vi "Build SPA query command substring.vi"(1 "Syntax":T1, 2 "Axes to query":string[](array[string]), 3 "Parameter number":i32[](array[numeric]), 6 "Parameter number (hex)":u32[](array[numeric]) format="%.0x", 7 "Parameter no. format \n(Decimal: FALSE)":bool) -> (14 "Command substring":string, 16 "Number of rows":u32)   [LabVIEW 2020]
doc: "This VI builds an SPA? Command substring. Axes and parameters are combined into a substring. Number of rows is size of Axes to query array. Sub-VI for SPA?.vi and SEP?.vi."
uses:
  Communication.llb/Syntax.ctl
panel:
  # "This vi builds a SPA? command substring. Axes and parameters are combined into a substring, depending on \"Parameter\nno. format\"."
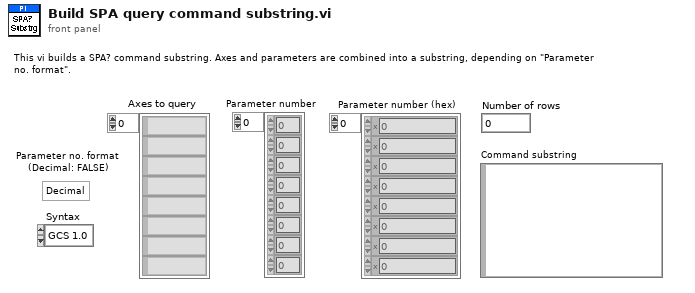
[diagram p1: front panel]
types:
  T1 = typedef "Syntax.ctl" = enum16{"GCS 1.0", "GCS 2.0", "GCS 3.0"}
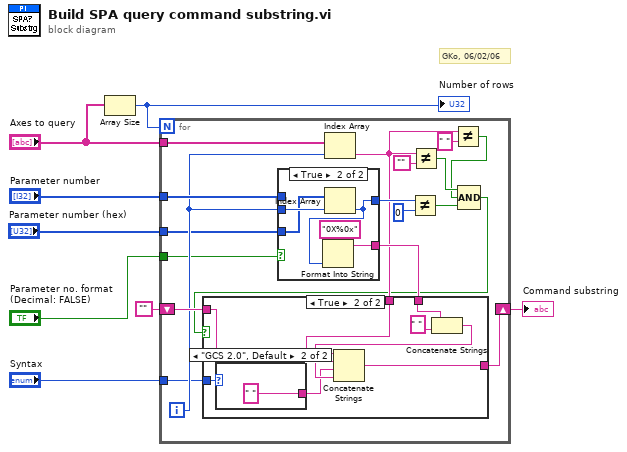
[diagram p0: block diagram]
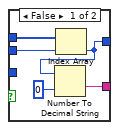
[diagram p2: hidden frame]
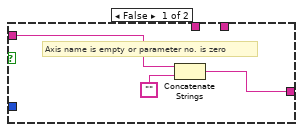
[diagram p3: hidden frame]
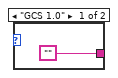
[diagram p4: hidden frame]
diagram:
  # "GKo, 06/02/06"
  n1 = Array Size(array="Axes to query") -> (size(s)=w8:i32)
  "Number of rows" <- w8
  n2 = for {
    N: w8 -> [_]
    shift-right: [w25] -> w6
    shift-left: "" -> [w26]
    tunnel: "Axes to query" -> [w24]
    tunnel: "Parameter number" -> [w23]
    tunnel: "Syntax" -> [w18]
    tunnel: "Parameter no. format \n(Decimal: FALSE)" -> [w10]
    tunnel: "Parameter number (hex)" -> [w9]
    i -> [w22]
    n3 = case shown="True" w10 {
      tunnel: w23 -> [w31 _]
      tunnel: w22 -> [w30 w36]
      tunnel: [w29 w35] -> w21
      tunnel: [w28 w34] -> w19
      tunnel: w9 -> [_ w33]
      frame False {
        n4 = Index Array(array=w31, index=w30) -> (element=w29:i32)
        n5 = Number To Decimal String(number=w29, width (-)=i16 0) -> (decimal integer string=w28:string)
      }
      frame True {
        n6 = Index Array(array=w33, index=w36) -> (element=w35:u32)
        n7 = Format Into String(format string="0X%0x" ("Format String"), w35) -> (resulting string=w34:string)  [unwired: 2 in, 1 out]
      }
    }
    n8 = Index Array(array=w24, index=w22) -> (element=w16:string)
    n9 = Not Equal?(x=w21, y=0 ("width (-)")) -> (x != y?=w12:bool)
    n10 = Not Equal?(x=w16, y="") -> (x != y?=w14:bool)
    n11 = Not Equal?(x=w16, y=" ") -> (x != y?=w13:bool)
    n12 = Compound Arithmetic op=AND(w14, w13, w12) -> (w11:bool)
    n13 = case shown="True" w11 {
      tunnel: w26 -> [w39 w47]
      tunnel: [w37 w46] -> w25
      tunnel: w16 -> [_ w45]
      tunnel: w19 -> [_ w44]
      tunnel: w18 -> [_ w42]
      frame False {
        # "Axis name is empty or parameter no. is zero"
        n14 = Concatenate Strings(w39, "") -> (w37:string)
      }
      frame True {
        n15 = case shown="\"GCS 2.0\", Default" w42 {
          tunnel: ["" " "] -> w40
          frame "GCS 1.0" {
          }
          frame "GCS 2.0", Default {
          }
        }
        n16 = Concatenate Strings(w44, " " ("Substring")) -> (w41:string)
        n17 = Concatenate Strings(w47, w45, w40, w41) -> (w46:string)
      }
    }
  }
  "Command substring" <- w6
